vi "SQL_OUT Stack Cmd.vi"(11 "parameter buffer":T1) -> (1 "结果":string, 2 "净重":string, 3 "连接的字符串":string)   [LabVIEW 2015]
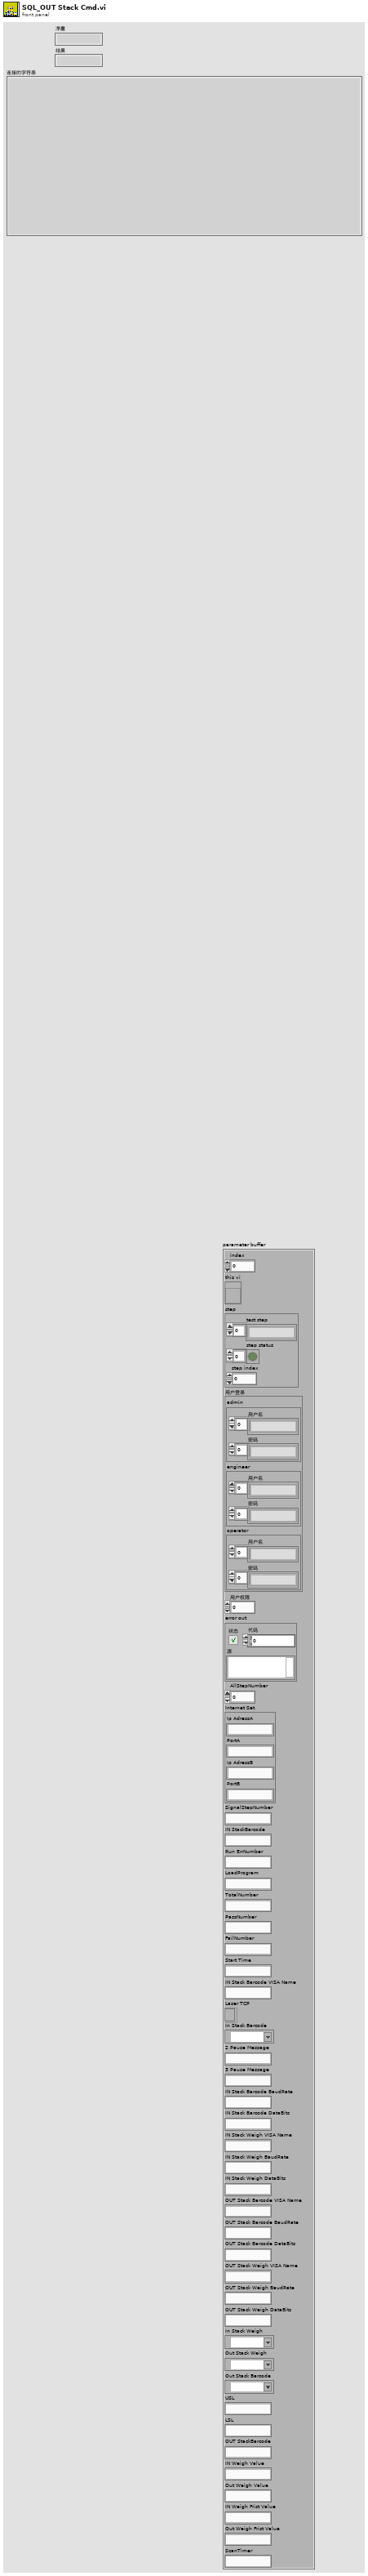
[diagram p1: front panel]
types:
  T1 = cluster{"index":i32, "this vi":refnum<vi>, "step":cluster{"test step":string[], "step status":bool[], "step index":i32}, "用户登录":cluster{"admin":cluster{"用户名":string[], "密码":string[]}, "engineer":cluster{"用户名":string[], "密码":string[]}, "operator":cluster{"用户名":string[], "密码":string[]}}, "用户权限":i32, "error out":errorcluster, "AllStepNumber":i32, "Internet Set":cluster{"Ip AdressA":string, "PortA":string, "Ip AdressB":string, "PortB":string}, "SignalStepNumber":string, "IN StackBarcode":string, "Run ErrNumber":string, "LoadProgram":string, "TotalNumber":string, "PassNumber":string, "FailNumber":string, "Start Time":string, "IN Stack Barcode VISA Name":string, "Laser TCP":refnum<k5>, "In Stack Barcode":refnum<visa-resource-name>, "2 Pause Message":string, "3 Pause Message":string, "IN Stack Barcode BaudRate":string, "IN Stack Barcode DataBits":string, "IN Stack Weigh VISA Name":string, "IN Stack Weigh BaudRate":string, "IN Stack Weigh DataBits":string, "OUT Stack Barcode VISA Name":string, "OUT Stack Barcode BaudRate":string, "OUT Stack Barcode DataBits":string, "OUT Stack Weigh VISA Name":string, "OUT Stack Weigh BaudRate":string, "OUT Stack Weigh DataBits":string, "In Stack Weigh":refnum<visa-resource-name>, "Out Stack Weigh":refnum<visa-resource-name>, "Out Stack Barcode":refnum<visa-resource-name>, "USL":string, "LSL":string, "OUT StackBarcode":string, "IN Weigh Value":string, "Out Weigh Value":string, "IN Weigh Frist Value":string, "Out Weigh Frist Value":string, "ScanTimer":string}
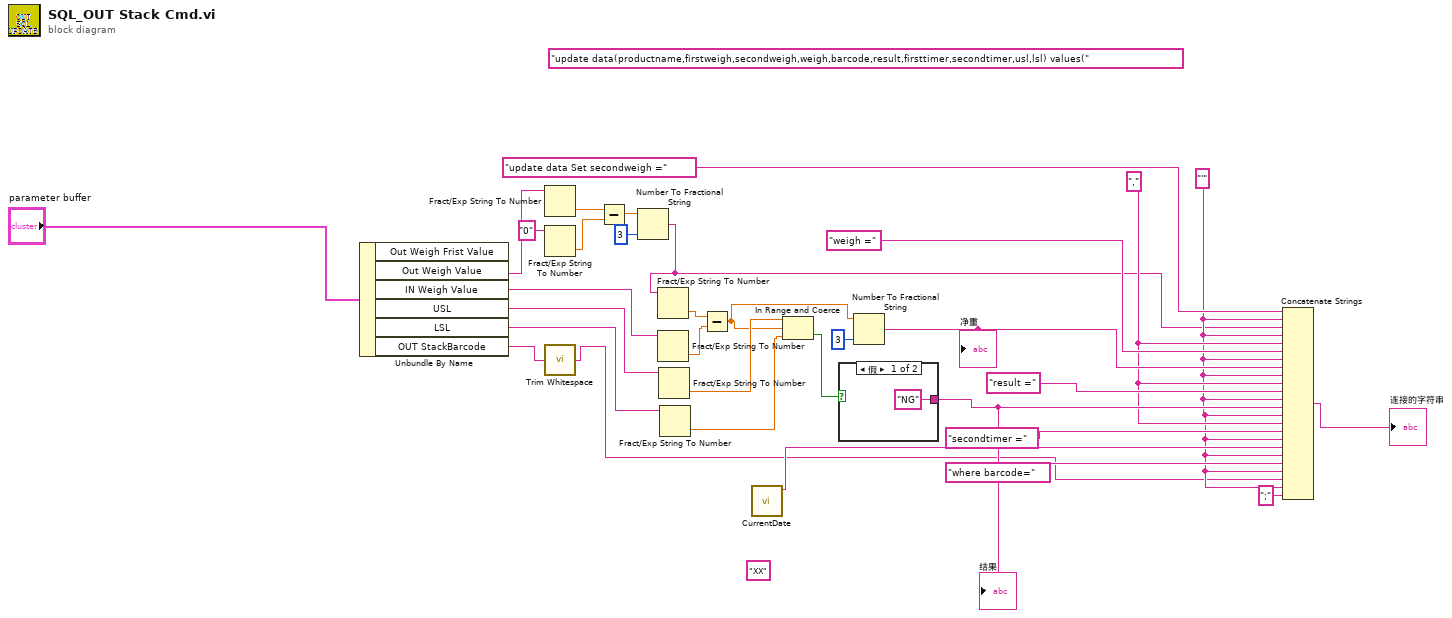
[diagram p0: block diagram]
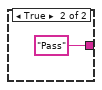
[diagram p2: hidden frame]
diagram:
  (unwired) "update data(productname,firstweigh,secondweigh,weigh,barcode,result,firsttimer,secondtimer,usl,lsl) values(" ("字符串")
  (unwired) "XX" ("字符串")
  w15 = ","
  w13 = "'"
  n1 = Unbundle By Name("parameter buffer") -> ("Out Weigh Value"=w10:string, "IN Weigh Value"=w30:string, "USL"=w11:string, "LSL"=w27:string, "OUT StackBarcode"=w2:string)  [unwired: 1 out]
  n2 = Fract/Exp String To Number(string=w10) -> (number=w9:dbl)  [unwired: 3 in, 1 out]
  n3 = Fract/Exp String To Number(string="0" ("字符串")) -> (number=w8:dbl)  [unwired: 3 in, 1 out]
  n4 = call <vilib>:"Trim Whitespace.vi"("string"=w2) -> ("trimmed string"=w1:string)  [unwired: 1 in]
  n5 = Subtract(x=w9, y=w8) -> (x-y=w7:dbl)
  n6 = Number To Fractional String(number=w7, precision (6)=i16 3 ("精度(6)")) -> (F-format string=w5:string)  [unwired: 2 in]
  n7 = Fract/Exp String To Number(string=w5) -> (number=w29:dbl)  [unwired: 3 in, 1 out]
  n8 = Fract/Exp String To Number(string=w30) -> (number=w28:dbl)  [unwired: 3 in, 1 out]
  n9 = Fract/Exp String To Number(string=w11) -> (number=w26:dbl)  [unwired: 3 in, 1 out]
  n10 = Fract/Exp String To Number(string=w27) -> (number=w25:dbl)  [unwired: 3 in, 1 out]
  n11 = Subtract(x=w29, y=w28) -> (x-y=w23:dbl)
  n12 = call "CurrentDate.vi"() -> ("当前日期时间"=w16:string)  [unwired: 11 in]
  n13 = In Range and Coerce(upper limit=w26, x=w23, lower limit=w25) -> (In Range?=w20:bool)  [unwired: 1 out]
  n14 = case shown="假" w20 {
    tunnel: ["NG" ("字符串") "Pass" ("字符串")] -> w18
    frame False {
    }
    frame True {
    }
  }
  "结果" <- w18
  n15 = Number To Fractional String(number=w23, precision (6)=i16 3 ("精度(6)")) -> (F-format string=w21:string)  [unwired: 2 in]
  "净重" <- w21
  n16 = Concatenate Strings("update data Set secondweigh =" ("字符串"), w13, w5, w13, w15, "weigh =" ("字符串"), w13, w21, w13, w15, "result =" ("字符串"), w13, w18, w13, w15, "secondtimer =" ("字符串"), w13, w16, w13, "where barcode=" ("字符串"), w13, w1, w13, ";" ("字符串")) -> (→"连接的字符串":string)
